vi "CustomShot.vi"(10 "HighShot":bool, 11 "Shoot":bool) -> (3 "All Driver Commands":T1)   [LabVIEW 2012]
uses:
  All_Commands.ctl
  Cirular Shooter/circular_shooter_commands.ctl
  Climber/Climber_Commands.ctl
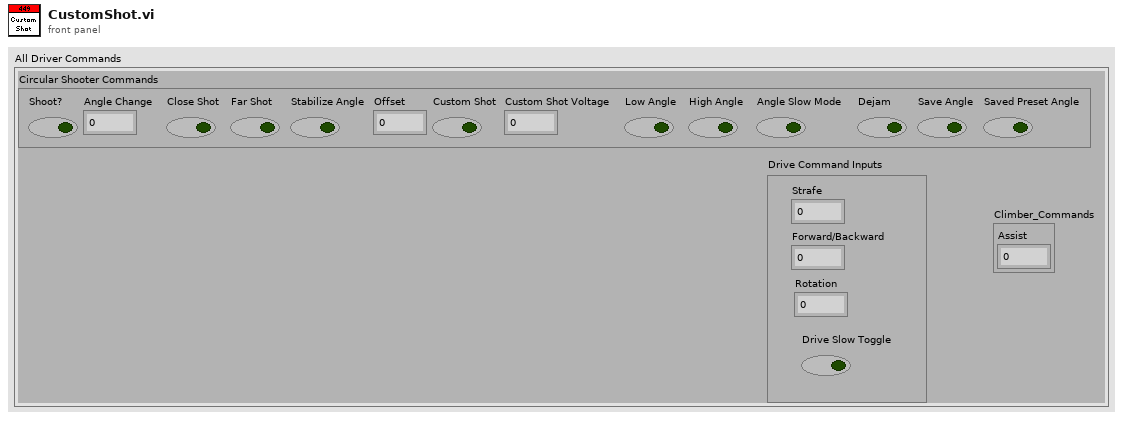
[diagram p1: front panel]
types:
  T1 = typedef "All_Commands.ctl" = cluster{"Circular Shooter Commands":T2, "Drive Command Inputs":cluster{"Strafe":dbl, "Forward/Backward":dbl, "Rotation":dbl, "Drive Slow Toggle":bool}, "Climber_Commands":T3}
  T2 = typedef "circular_shooter_commands.ctl" = cluster{"Shoot?":bool, "Angle Change":dbl, "Close Shot":bool, "Far Shot":bool, "Stabilize Angle ":bool, "Offset":dbl, "Custom Shot":bool, "Custom Shot Voltage":dbl, "Low Angle":bool, "High Angle":bool, "Angle Slow Mode":bool, "Dejam":bool, "Save Angle":bool, "Saved Preset Angle":bool}
  T3 = typedef "Climber_Commands.ctl" = cluster{"Assist":dbl}
  T4 = cluster{"Strafe":dbl, "Forward/Backward":dbl, "Rotation":dbl, "Drive Slow Toggle":bool}
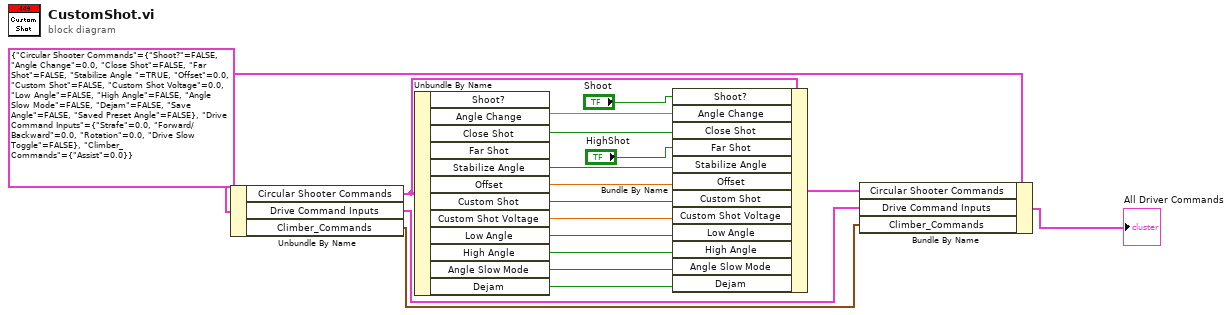
[diagram p0: block diagram]
diagram:
  w5 = T1 {"Circular Shooter Commands"={"Shoot?"=FALSE, "Angle Change"=0.0, "Close Shot"=FALSE, "Far Shot"=FALSE, "Stabilize Angle "=TRUE, "Offset"=0.0, "Custom Shot"=FALSE, "Custom Shot Voltage"=0.0, "Low Angle"=FALSE, "High Angle"=FALSE, "Angle Slow Mode"=FALSE, "Dejam"=FALSE, "Save Angle"=FALSE, "Saved Preset Angle"=FALSE}, "Drive Command Inputs"={"Strafe"=0.0, "Forward/Backward"=0.0, "Rotation"=0.0, "Drive Slow Toggle"=FALSE}, "Climber_Commands"={"Assist"=0.0}} ("All Driver Commands")
  n1 = Unbundle By Name(w5) -> ("Circular Shooter Commands"=w18:T2, "Drive Command Inputs"=w3:T4, "Climber_Commands"=w2:T3)
  n2 = Unbundle By Name(w18) -> ("Angle Change"=w17:dbl, "Close Shot"=w14:bool, "Stabilize Angle"=w13:bool, "Offset"=w12:dbl, "Custom Shot"=w11:bool, "Custom Shot Voltage"=w10:dbl, "Low Angle"=w9:bool, "High Angle"=w8:bool, "Angle Slow Mode"=w7:bool, "Dejam"=w6:bool)  [unwired: 2 out]
  n3 = Bundle By Name(cluster=w18, "Shoot?"="Shoot", "Angle Change"=w17, "Close Shot"=w14, "Far Shot"="HighShot", "Stabilize Angle"=w13, "Offset"=w12, "Custom Shot"=w11, "Custom Shot Voltage"=w10, "Low Angle"=w9, "High Angle"=w8, "Angle Slow Mode"=w7, "Dejam"=w6) -> (w4:T2)
  n4 = Bundle By Name(cluster=w5, "Circular Shooter Commands"=w4, "Drive Command Inputs"=w3, "Climber_Commands"=w2) -> (→"All Driver Commands":T1)
